vi "Set_Rois.vi"(8 "error in":errorcluster, 10 "PicamROI":T1, 11 "camera handle in":u64) -> (0 "error out":errorcluster, 3 "camera handle out":u64)   [LabVIEW 2014, in "PICam.lvlib"]
doc: "Picam_SetParameterRoisValue() configures an Rois parameter to a specified value\nduring camera setup.\n\nIn this VI implementation we only want to specify a single ROI, so the input is a single ROI cluster!"
uses:
  PICam.lvlib
  Ctrls/PicamROI.ctl
  Program Files/Princeton Instruments/PICam/Runtime/Picam32.dll
panel:
  out "roid":cluster{"roi (U32)":u32, "count (I32)":i32}
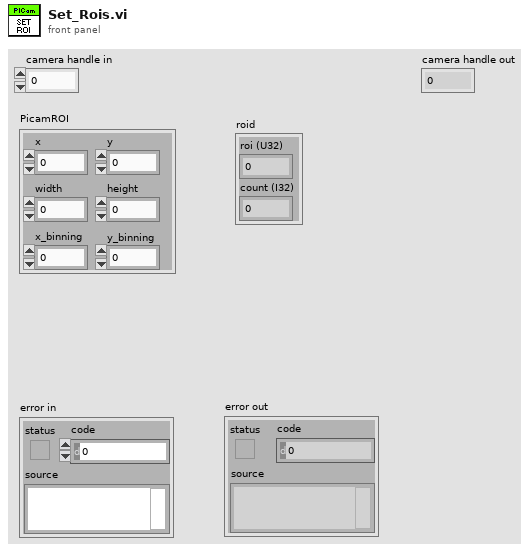
[diagram p1: front panel]
types:
  T1 = typedef "PICam.lvlib/PicamROI.ctl" = cluster{"x":i32, "width":i32, "x_binning":i32, "y":i32, "height":i32, "y_binning":i32}
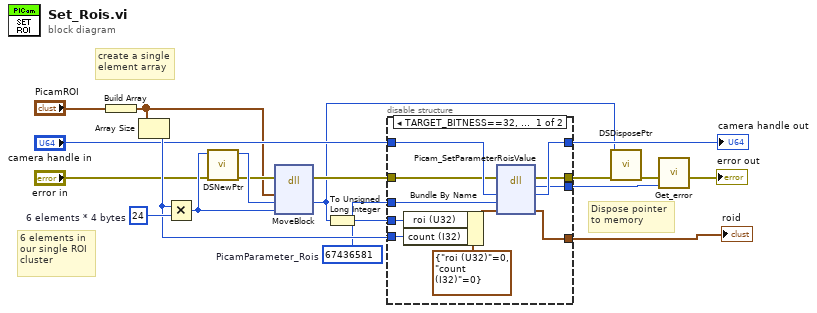
[diagram p0: block diagram]
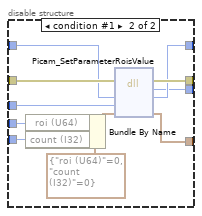
[diagram p2: hidden frame]
diagram:
  w18 = 24  # 6 elements * 4 bytes
  w11 = u32 67436581  # PicamParameter_Rois
  # "create a single\nelement array"
  # "6 elements in\nour single ROI\ncluster"
  # "Dispose pointer\nto memory"
  n1 = Build Array("PicamROI") -> (w7:T1[])
  n2 = Array Size(array=w7) -> (size(s)=w14:i32)
  n3 = Multiply(x=w14, y=w18) -> (x*y=w17:i32)
  n4 = call <vilib>:"DSNewPtr.vi"("error in (no error)"="error in", "Size"=w17) -> ("error out"=w16:errorcluster, "Pointer"=w19:u64)  [unwired: 8 in]
  n5 = dll-call lib="LabVIEW" fn="MoveBlock"(error in=w16, "src"=w7, "dst"=w19, "size"=w17) -> (error out=w15:errorcluster, "dst"=w6:u64)  [unwired: 5 in, 1 out]
  n6 = To Unsigned Long Integer(number=w6) -> (unsigned 32bit integer=w1:u32)
  n7 = disable-structure shown="TARGET_BITNESS==32, Default" {
    disable-tunnel: "camera handle in" -> [w28 w38]
    disable-tunnel: w1 -> [w24 w36]
    disable-tunnel: w15 -> [w27 w41]
    disable-tunnel: [w26 w37] -> w12
    disable-tunnel: w11 -> [w25 w32]
    disable-tunnel: [w23 w40] -> w13
    disable-tunnel: w14 -> [w22 w35]
    disable-tunnel: [w21 w34] -> w5
    disable-tunnel: [w20 w31] -> w2
    frame condition #0 (active) {
      n8 = Bundle By Name(cluster=cluster{"roi (U32)":u32, "count (I32)":i32} {"roi (U32)"=0, "count (I32)"=0}, "roi (U32)"=w24, "count (I32)"=w22) -> (w29:cluster{"roi (U32)":u32, "count (I32)":i32})
      n9 = dll-call lib="C:/Program Files/Princeton Instruments/PICam/Runtime/picam32.dll" fn="Picam_SetParameterRoisValue"(error in=w27, "handle"=w28, "param"=w25, "roid"=w29) -> (error out=w23:errorcluster, "return type"=w21:i32, "handle"=w26:u64, "roid"=w20:cluster{"roi (U32)":u32, "count (I32)":i32})  [unwired: 3 in, 1 out]
    }
    frame condition #1 {
      n10 = Bundle By Name(cluster=cluster{"roi (U64)":u64, "count (I32)":i32} {"roi (U64)"=0, "count (I32)"=0}, "roi (U64)"=w36, "count (I32)"=w35) -> (w39:cluster{"roi (U64)":u64, "count (I32)":i32})
      n11 = dll-call lib="C:/Program Files/Princeton Instruments/PICam/Runtime/picam32.dll" fn="Picam_SetParameterRoisValue"(error in=w41, "handle"=w38, "param"=w32, "roid"=w39) -> (error out=w40:errorcluster, "return type"=w34:i32, "handle"=w37:u64, "roid"=w31:cluster{"roi (U64)":u64, "count (I32)":i32})  [unwired: 3 in, 1 out]
    }
  }
  "camera handle out" <- w12
  "roid" <- w2
  n12 = call <vilib>:"DSDisposePtr.vi"("error in (no error)"=w13, "Pointer"=w6) -> ("error out"=w4:errorcluster)  [unwired: 9 in]
  n13 = call "Get_error.vi"("PICam_Error"=w5, "error in (no error)"=w4) -> ("error out"=→"error out":errorcluster)  [unwired: 9 in]
